vi "While.vi"() -> ()   [LabVIEW 2018]
panel:
  out "숫자형":i32
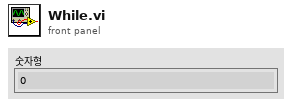
[diagram p1: front panel]
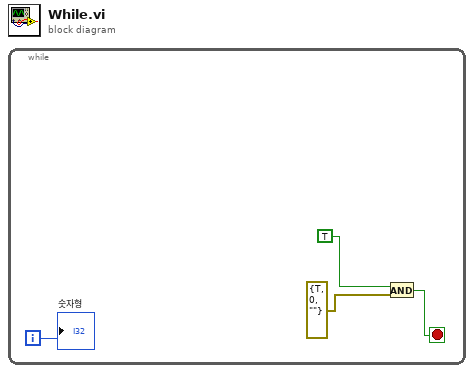
[diagram p0: block diagram]
diagram:
  n1 = while {
    i -> [w4]
    stop <- w3 stop-if-true
    n2 = And(x=TRUE, y=errorcluster {"status"=TRUE, "code"=0, "source"=""} ("에러 상수")) -> (x .and. y?=w3:bool)
    "숫자형" <- w4
  }
